vi "Upload to ADAM Server.vi"() -> (5 "Plug in titles":string[](array[string]), 7 "Plug in values":string[](array[string]))   [LabVIEW 2020]
uses:
  Globals/Meas_global.vi
  Globals/Preference_global.vi
panel:
  out "Values":dbl[](array[numeric])
  out "Array":string[](array[string])
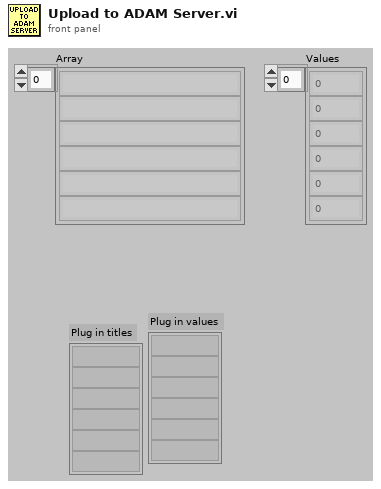
[diagram p1: front panel]
types:
  T1 = typedef "Analysis_info_cluster.ctl" = cluster{"Colour":u32, "Inst type":T2, "Inst name":string, "Symbol":string, "Code name":string, "Extra Info":string, "Inst Array":T3, "Extra Titles":string[], "Extra Values":string[], "U":dbl, "u^2":dbl, "u^3":dbl, "u^4":dbl, "Skew_u":dbl, "Kurt_u":dbl, "Sd Error in Mean":dbl, "% u'/U":dbl, "X":dbl, "Y":dbl, "Z":dbl, "Timescale integral Estimate":dbl, "Sd Error in Variance":dbl, "Calib File":path, "Calib Constants":dbl[], "Output Position":bool, "Stats":enum16{"None", "Basic", "Full"}, "Av Sampling Rate":dbl, "Av No of Samples":dbl, "Total Meas Time (s)":dbl, "ADAM Ch Name":string, "Max value":dbl, "Min value":dbl, "Req Sample Rate Hz":dbl, "Sync Delay Time (s)":dbl, "Ch No":i16, "Device":string, "Use Latest Calib":bool, "Port":string, "Metadata Ch Names":string[], "Metadata Ch Values":string[], "Label":string}
  T2 = typedef "Inst_type.ctl" = enum16{"Raw voltage", "Raw with zero offsetting", "Propeller anemometer", "Pressure Transducer", "Pitot-static tube", "Hot wire", "Cross wire 1", "Cross wire 2", "Generic Linear", "Generic Polynomial", "Generic BackPoly", "Fast FID", "Thermocouple", "Cold wire", "Pulsed Wire", "LDA Vel", "LDA Tran time", "LDA Arr time", "Microphone"}
  T3 = typedef "Instrument_Array.ctl" = enum16{"PWA", "LDA", "Analogue"}
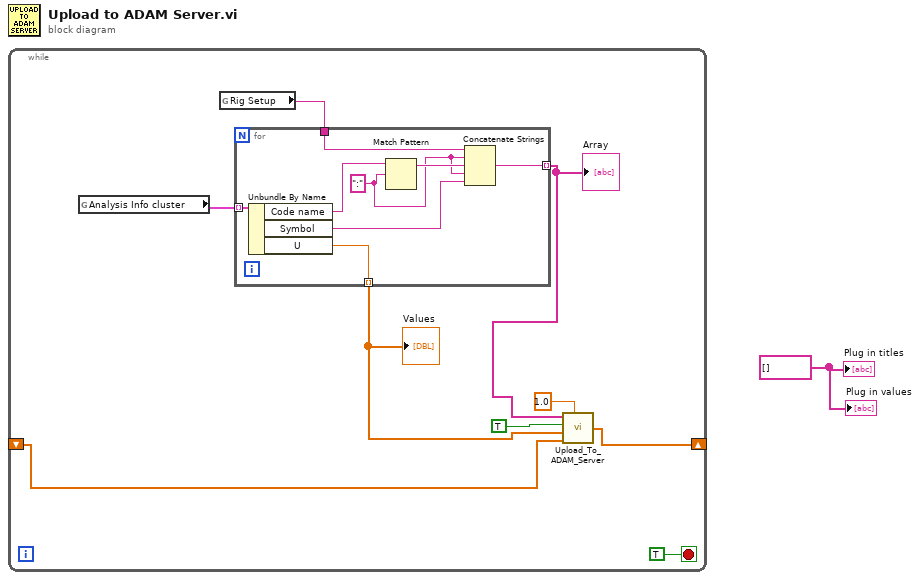
[diagram p0: block diagram]
diagram:
  w1 = string[] [] ("Plug in titles")
  n1 = while {
    shift-right: [w4] -> _
    shift-left: _ -> [w3]
    stop <- TRUE stop-if-true
    n2 = global read "Meas_global.vi" "Analysis Info cluster"() -> (w10:T1[])
    n3 = global read "Preference_global.vi" "Rig Setup"() -> (w9:string)
    n4 = for {
      tunnel: w10 -> [w18] mode=indexing
      tunnel: w9 -> [w16]
      tunnel: [w12] -> w6 mode=indexing
      tunnel: [w11] -> w5 mode=indexing
      w14 = ":" ("regular expression")
      n5 = Unbundle By Name(w18) -> ("Code name"=w17:string, "Symbol"=w13:string, "U"=w11:dbl)
      n6 = Match Pattern(string=w17, regular expression=w14) -> (before substring=w15:string)  [unwired: 1 in, 3 out]
      n7 = Concatenate Strings(w16, w14, w15, w14, w13) -> (w12:string)
    }
    "Array" <- w6
    "Values" <- w5
    n8 = call "Upload_To_ADAM_Server.vi"("Averaging Period (s)"=1.0, "Shift In"=w3, "Channel Values"=w5, "Give Variance"=TRUE, "Channel Names"=w6) -> ("Shift Out"=w4:dbl[])  [unwired: 1 in]
  }
  "Plug in values" <- w1
  "Plug in titles" <- w1
